vi "Create Slots.vi"(7 "error in":errorcluster, 8 "EtherCAT?":bool, 9 "Num Slots":i32=8, 10 "Item Ref In":T1 format="%.0x") -> (0 "error out":errorcluster, 1 "user variables ref":T1 format="%.0x", 2 "slot refs":T1[](array[typedef]) format="%.0x", 3 "Item Ref out":T1 format="%.0x")   [LabVIEW 2019, in "SEECD System Explorer.lvlib"]
uses:
  SEECD System Explorer.lvlib
  <vilib>/NI VeriStand/Custom Device API/Custom Device Item Ref.ctl
  Includes/Modules.lvlibp/RSI Module/Module Models.ctl
  Includes/Modules.lvlibp/RSI Module/Slot Settings.ctl
  Shared/Globals/Scan Engine GUIDs.vi
  Shared/Globals/Property Strings.vi
  Shared/Globals/String Constants.vi
  Includes/Modules.lvlibp/RSI Module/Class Property Strings.vi
  <vilib>/NI VeriStand/Custom Device API/Custom Device API.lvlib
  Shared/SEECD Shared.lvlib
  Includes/Modules.lvlibp/RSI Module/RSI Module.lvclass
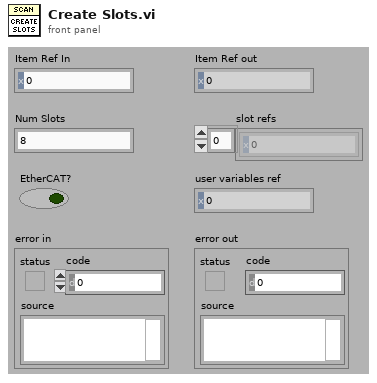
[diagram p1: front panel]
types:
  T1 = typedef "Custom Device API.lvlib/Custom Device Item Ref.ctl" = u64
  T2 = typedef "Modules.lvlibp/RSI Module.lvclass/Slot Settings.ctl" = cluster{"Slot":u32, "EtherCAT?":bool}
  T3 = typedef "Modules.lvlibp/RSI Module.lvclass/Module Models.ctl" = enum16{"Empty", "NI 9201", "NI 9203", "NI 9205", "NI 9206", "NI 9207", "NI 9208", "NI 9209", "NI 9210", "NI 9211", "NI 9212", "NI 9213", "NI 9214", "NI 9215", "NI 9216", "NI 9217", "NI 9219", "NI 9220", "NI 9221", "NI 9222", "NI 9223", "NI 9224", "NI 9225", "NI 9226", "NI 9227", "NI 9228", "NI 9229", "NI 9233", "NI 9234", "NI 9235", "NI 9236", "NI 9237", "NI 9239", "NI 9242", "NI 9244", "NI 9253", "NI 9263", "NI 9264", "NI 9265", "NI 9266", "NI 9269", "NI 9344", "NI 9350", "NI 9375", "NI 9401", "NI 9402", "NI 9403", "NI 9411", "NI 9421", "NI 9422", "NI 9423", "NI 9425", "NI 9426", "NI 9435", "NI 9436", "NI 9437", "NI 9472", "NI 9474", "NI 9475", "NI 9476", "NI 9477", "NI 9478", "NI 9481", "NI 9482", "NI 9485"}
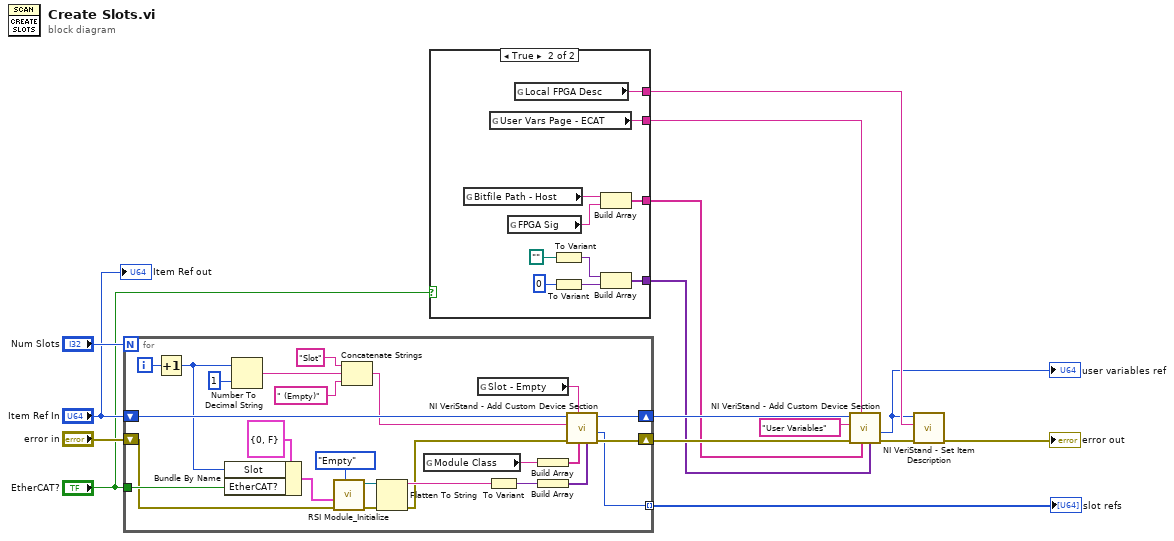
[diagram p0: block diagram]
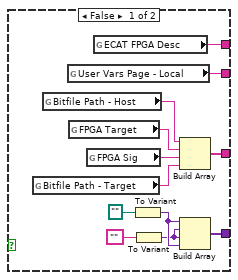
[diagram p2: hidden frame]
diagram:
  n1 = for {
    N: "Num Slots" -> [_]
    tunnel: "EtherCAT?" -> [w26]
    shift-right: [w35] -> w12
    shift-left: "error in" -> [w22]
    shift-right: [w34] -> w13
    shift-left: "Item Ref In" -> [w40]
    tunnel: [w16] -> w1 mode=indexing
    i -> [w37]
    n2 = Increment(x=w37) -> (x+1=w31:i32)
    n3 = Bundle By Name(cluster=T2 {"Slot"=0, "EtherCAT?"=FALSE} ("Slot Settings"), "Slot"=w31, "EtherCAT?"=w26) -> (w20:T2)
    n4 = Number To Decimal String(number=w31, width (-)=i16 1) -> (decimal integer string=w39:string)
    n5 = call "RSI Module_Initialize.vi"("Module Model"=Module_Models."Empty" ("Module"), "error in (no error)"=w22, "Slot Settings"=w20) -> ("error out"=w21:errorcluster, "RSI Module out"=w17:refnum<class "RSI Module.lvclass">)  [unwired: 7 in]
    n6 = Concatenate Strings("Slot" ("string"), w39, " (Empty)" ("Section Name")) -> (w36:string)
    n7 = Flatten To String(anything=w17, error in (no error)=w21) -> (data string=w25:string, error out=w24:errorcluster)  [unwired: 2 in, 1 out]
    n8 = global read "Class Property Strings.vi" "Module Class"() -> (w23:string)
    n9 = global read "Scan Engine GUIDs.vi" "Slot - Empty"() -> (w27:string)
    n10 = To Variant(anything=w25) -> (Variant=w32:variant)
    n11 = Build Array(w23) -> (w29:string[])
    n12 = Build Array(w32) -> (w33:variant[])
    n13 = call <vilib>:"NI VeriStand - Add Custom Device Section.vi"("Property Values"=w33, "Property names"=w29, "GUID (Default Section)"=w27, "error in (no error)"=w24, "Section Name"=w36, "Parent Ref in"=w40) -> ("error out"=w35:errorcluster, "Section Ptr"=w16:T1, "Parent Ref out"=w34:T1)  [unwired: 2 in, 1 out]
  }
  "slot refs" <- w1
  n14 = case shown="True" "EtherCAT?" {
    tunnel: [w44 w54] -> w9
    tunnel: [w43 w55] -> w8
    tunnel: [w42 w56] -> w10
    tunnel: [w41 w53] -> w5
    frame False {
      n15 = global read "Property Strings.vi" "Bitfile Path - Target"() -> (w48:string)
      n16 = global read "Property Strings.vi" "Bitfile Path - Host"() -> (w51:string)
      n17 = global read "Scan Engine GUIDs.vi" "User Vars Page - Local"() -> (w42:string)
      n18 = global read "Property Strings.vi" "FPGA Target"() -> (w50:string)
      n19 = global read "Property Strings.vi" "FPGA Sig"() -> (w49:string)
      n20 = global read "String Constants.vi" "ECAT FPGA Desc"() -> (w41:string)
      n21 = To Variant(anything=path "") -> (Variant=w47:variant)
      n22 = To Variant(anything="") -> (Variant=w45:variant)
      n23 = Build Array(w51, w50, w49, w48) -> (w43:string[])
      n24 = Build Array(w47, w45, w45, w47) -> (w44:variant[])
    }
    frame True {
      n25 = global read "Property Strings.vi" "Bitfile Path - Host"() -> (w58:string)
      n26 = global read "Scan Engine GUIDs.vi" "User Vars Page - ECAT"() -> (w56:string)
      n27 = global read "Property Strings.vi" "FPGA Sig"() -> (w57:string)
      n28 = global read "String Constants.vi" "Local FPGA Desc"() -> (w53:string)
      n29 = To Variant(anything=path "") -> (Variant=w60:variant)
      n30 = To Variant(anything=u32 0 ("ModuleIdent (ECAT)")) -> (Variant=w59:variant)
      n31 = Build Array(w58, w57) -> (w55:string[])
      n32 = Build Array(w60, w59) -> (w54:variant[])
    }
  }
  n33 = call <vilib>:"NI VeriStand - Add Custom Device Section.vi"("Property Values"=w9, "Property names"=w8, "GUID (Default Section)"=w10, "error in (no error)"=w12, "Section Name"="User Variables", "Parent Ref in"=w13) -> ("error out"=w4:errorcluster, "Section Ptr"=w3:T1)  [unwired: 2 in, 2 out]
  "user variables ref" <- w3
  n34 = call <vilib>:"NI VeriStand - Set Item Description.vi"("error in (no error)"=w4, "Description"=w5, "Item Ref in"=w3) -> ("error out"=→"error out":errorcluster)  [unwired: 6 in, 2 out]
  "Item Ref out" <- "Item Ref In"
